vi "GUI_HTU_Vacuum.vi"() -> ()   [LabVIEW 2020]
uses:
  Shared/GUI_Template/GUI_master/tcp_new_data_event.ctl
  Shared/GUI_Template/GUI_master/tcp new data cluster.ctl
panel:
  out "AI_mean.Channel 3::1":dbl caption="Energy (nJ)" min=0.0 max=0.0 format="%.3f"
  out "AI_mean.Channel 2::1":dbl caption="Energy (nJ)" min=0.0 max=0.0 format="%.3f"
  out "highPressure 4":bool=TRUE
  out "highPressure 3":bool=TRUE
  out "Compressor":dbl format="%_6g"
  out "OAP":dbl
  out "highPressure 2":bool=TRUE
  out "highPressure":bool=TRUE
  in  "GUIdevice 2":string="U_DG645_ShotControl"
  out "TargetChamberP":dbl format="%_6g"
  out "UndulatorP":dbl
  out "AI_mean.Channel 1::1":dbl caption="Energy (nJ)" min=0.0 max=0.0 format="%.3f"
  out "AI_mean.Channel 0::1":dbl caption="Energy (nJ)" min=0.0 max=0.0 format="%.3f"
  in  "UDP error message":string
  in  "GUIdevice 1":string="U_VacuumGauge"
  out "error IO 2":errorcluster
  out "tcp data event":T1
  in  "stop":bool
  out "Chart":T2(graph)
  # "HTU Vacuum"
  # "Pressure (Torr)"
  # "Comp chamber"
  # "OAP chamber"
  # "Target chamber"
  # "A-cave"
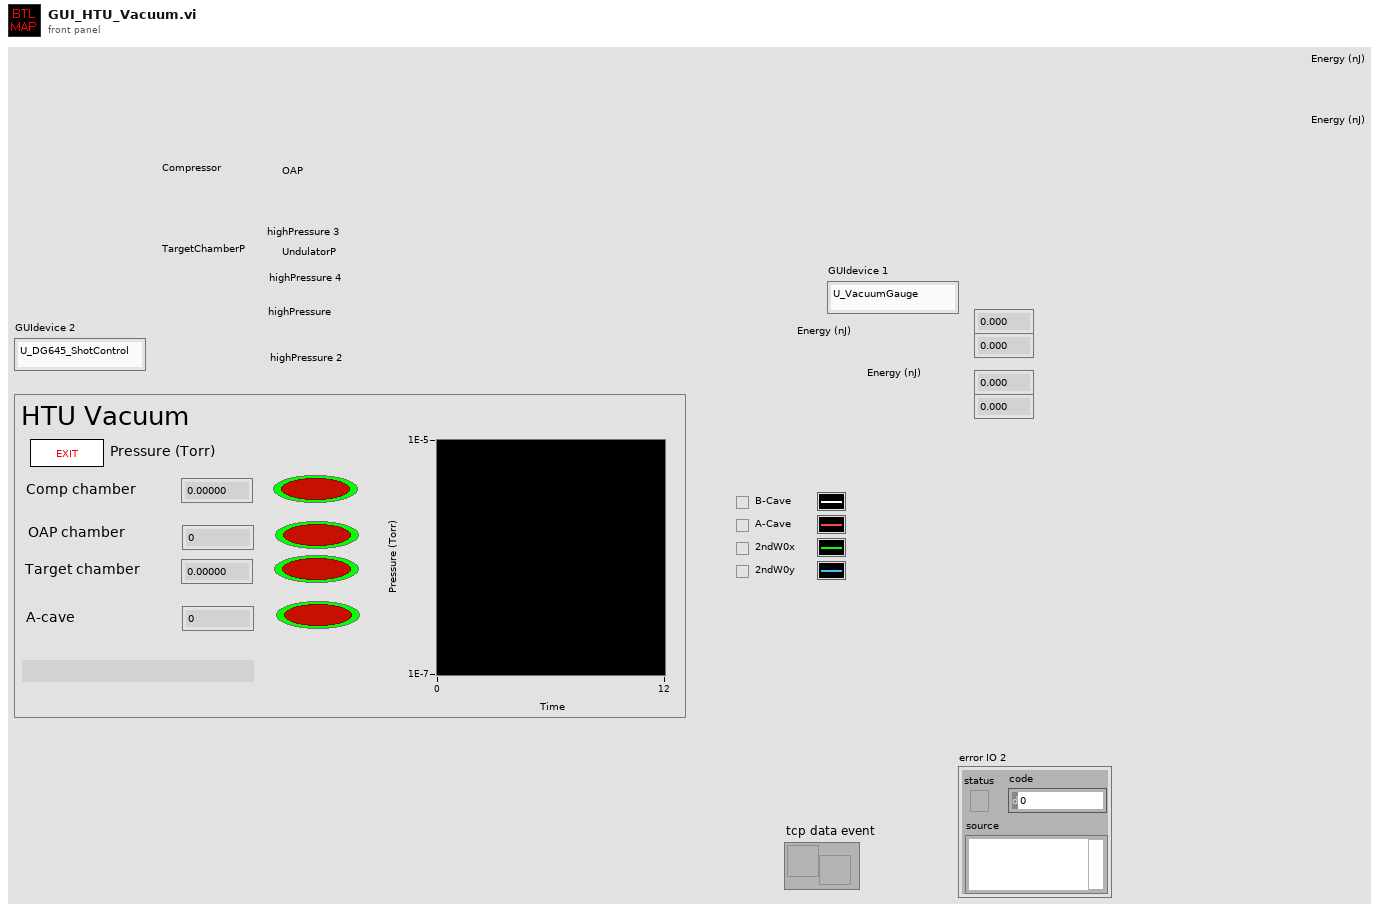
[diagram p1: front panel]
types:
  T1 = typedef "tcp_new_data_event.ctl" = refnum<user-event>
  T2 = cluster{"output variable":dbl, "output variable":dbl, "output variable":dbl, "output variable":dbl}
  T3 = typedef "tcp new data cluster.ctl" = cluster{"EventEnum":enum16{"new data", "connection status update"}, "Device name":string}
  T4 = enum32{"invalid app kind", "Development System", "Run Time System", "Student Edition", "Embedded LabVIEW", "Evaluation", "Custom"}
  T5 = enum32{"Invalid", "Standard", "Closed", "Hidden", "Minimized", "Maximized"}
  T6 = cluster{"Core":cluster{"Current VI Reference":refnum<vi>, "Close Panel on Exit?":bool}, "last chart update tck":i32, "TargetChamber":dbl, "Undulator":dbl, "CompressorChamber":dbl, "OAPChamber":dbl}
  T7 = cluster{"Current VI Reference":refnum<vi>, "Close Panel on Exit?":bool}
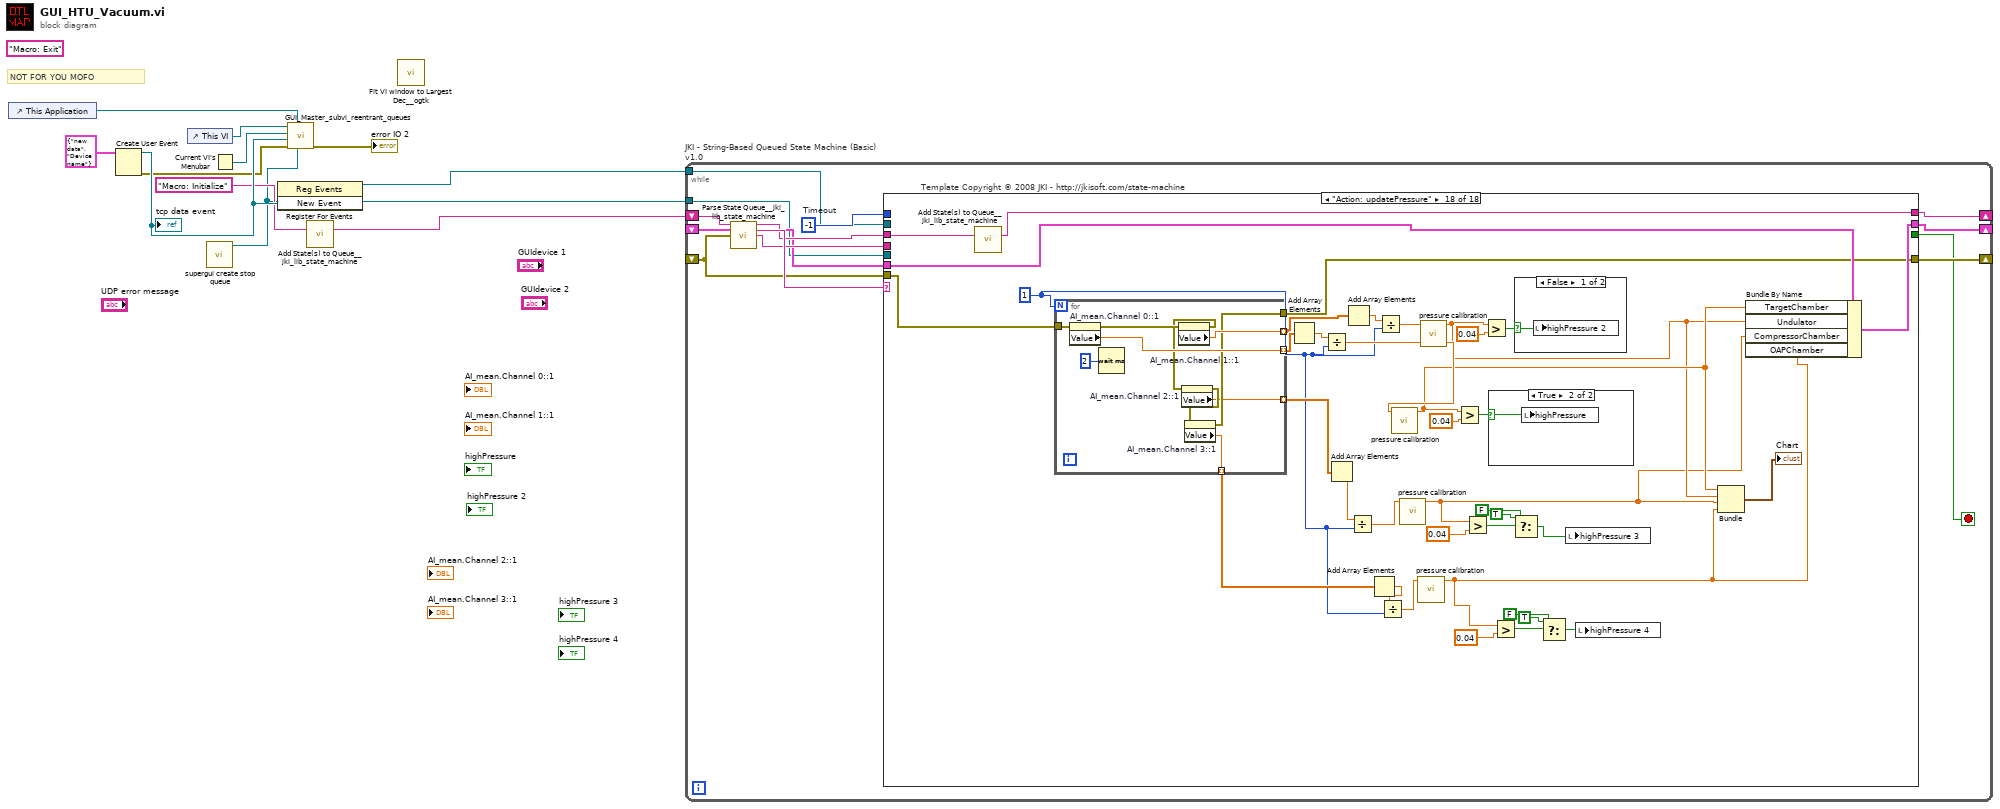
[diagram p0: block diagram]
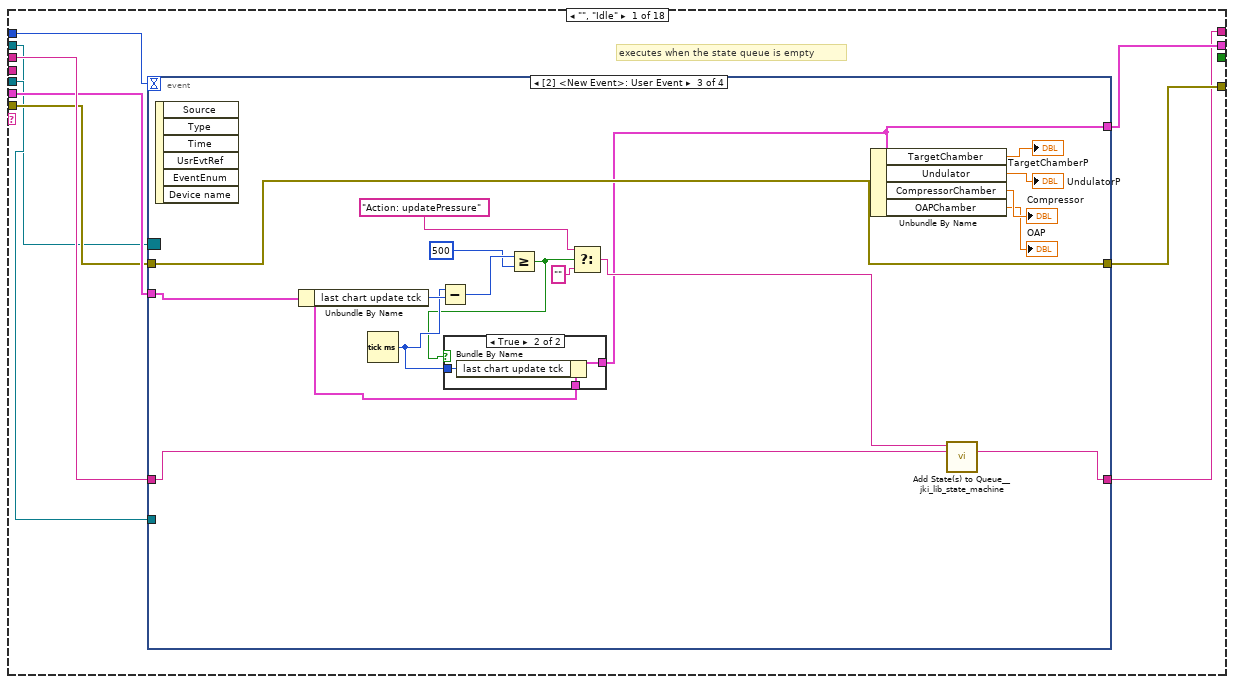
[diagram p2: hidden frame]
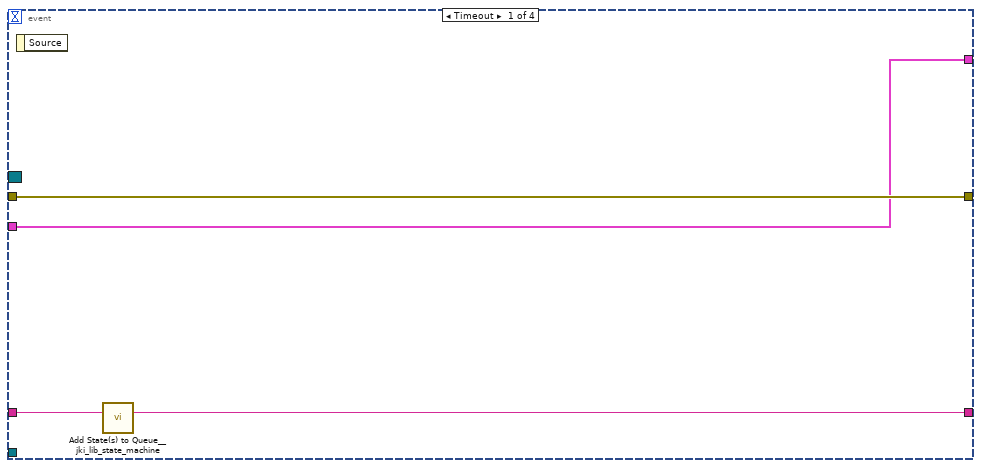
[diagram p3: hidden frame]
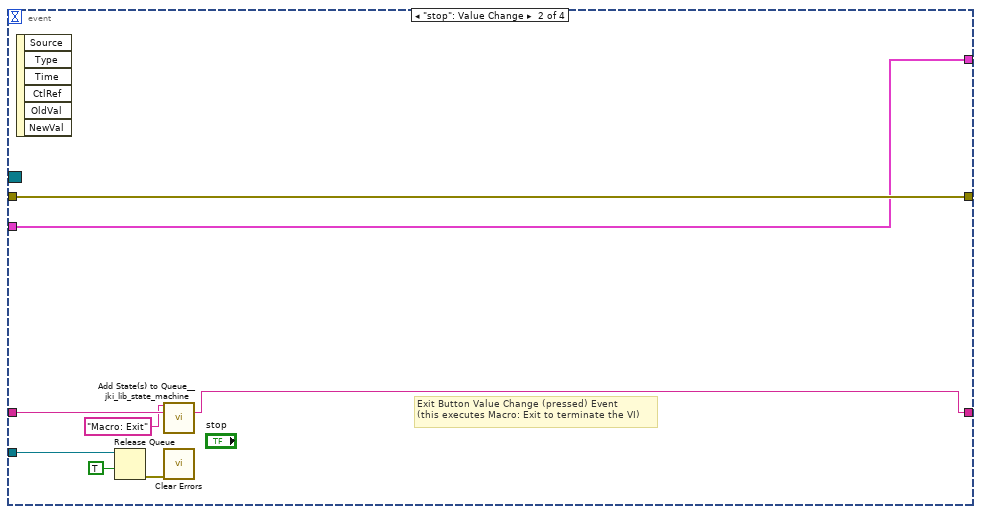
[diagram p4: hidden frame]
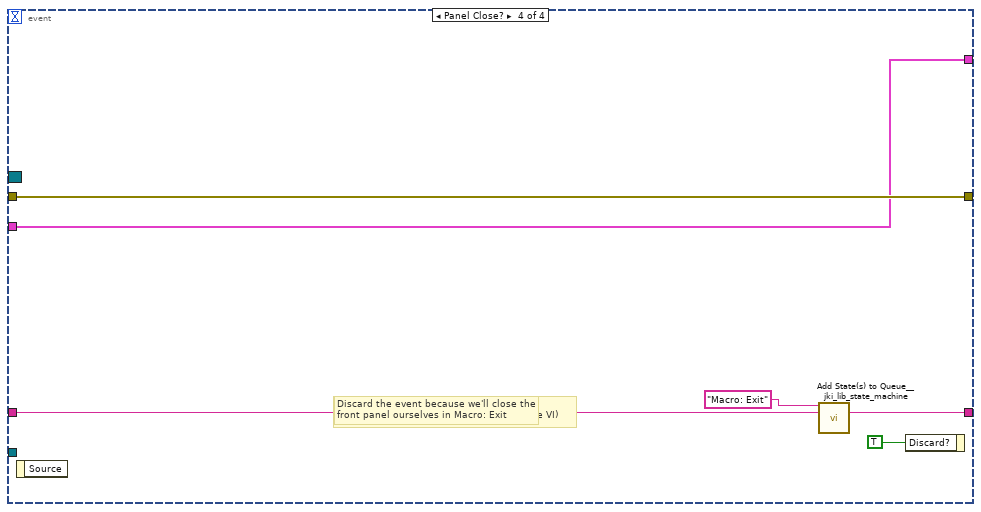
[diagram p6: hidden frame]
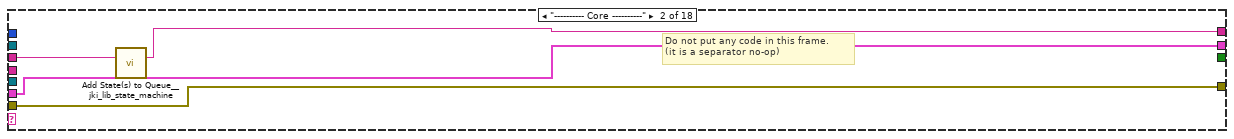
[diagram p7: hidden frame]
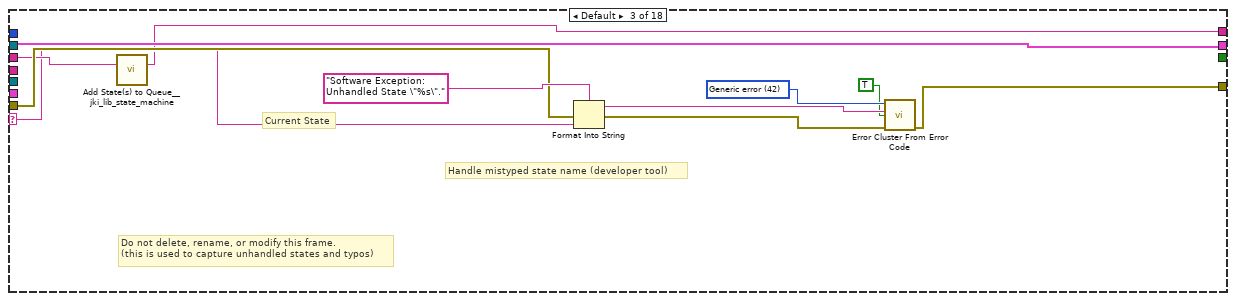
[diagram p8: hidden frame]
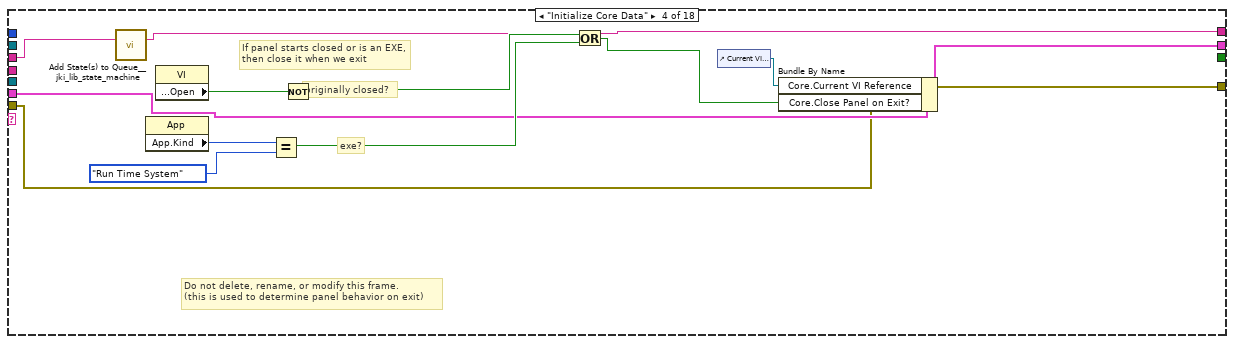
[diagram p9: hidden frame]
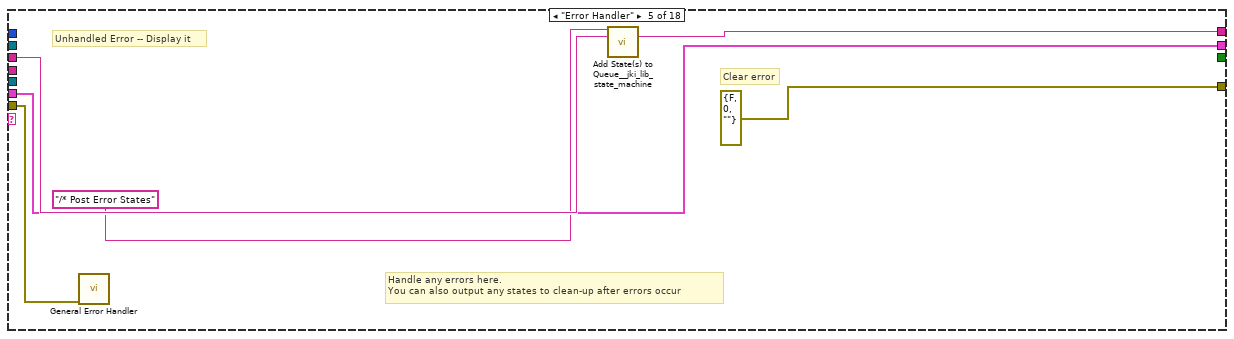
[diagram p10: hidden frame]
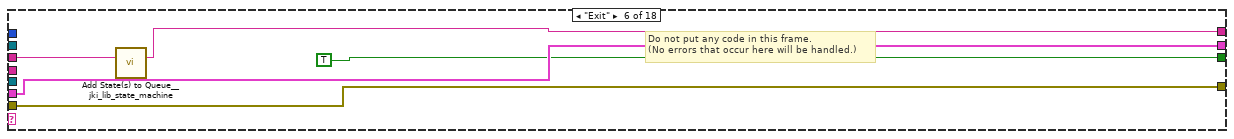
[diagram p11: hidden frame]
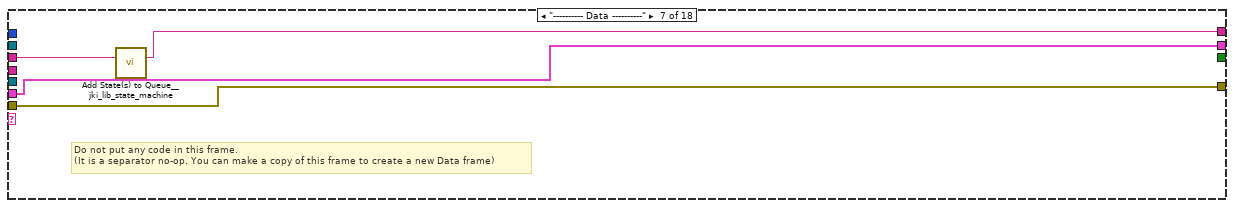
[diagram p12: hidden frame]
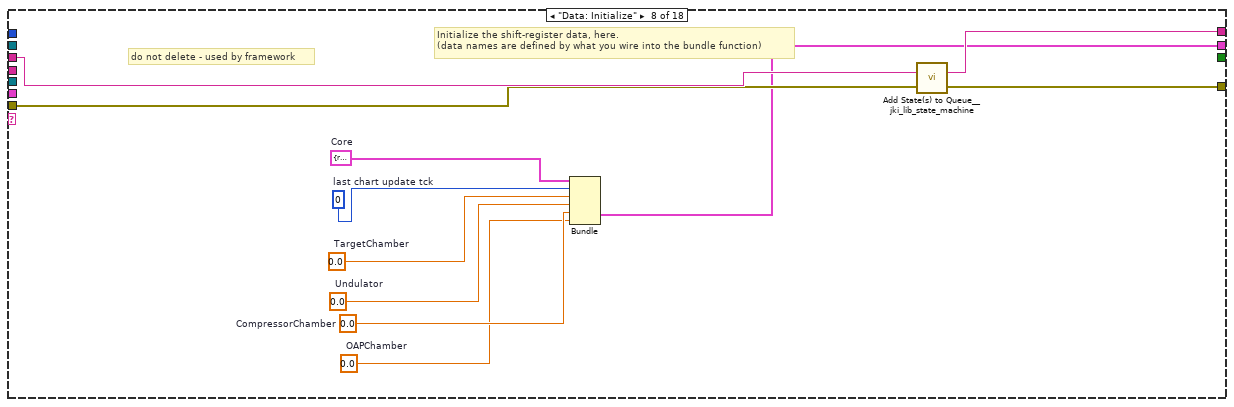
[diagram p13: hidden frame]
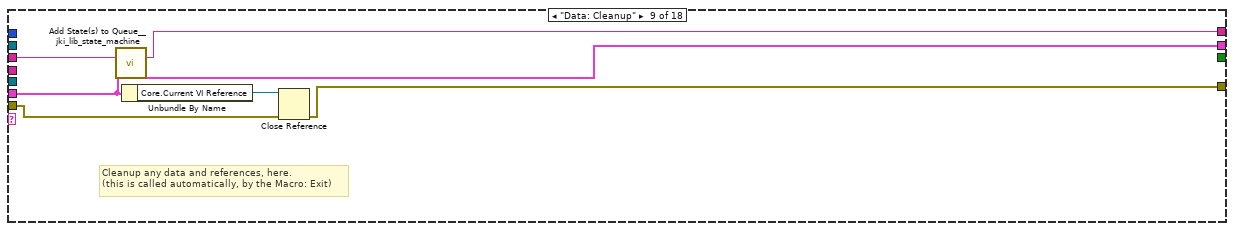
[diagram p14: hidden frame]
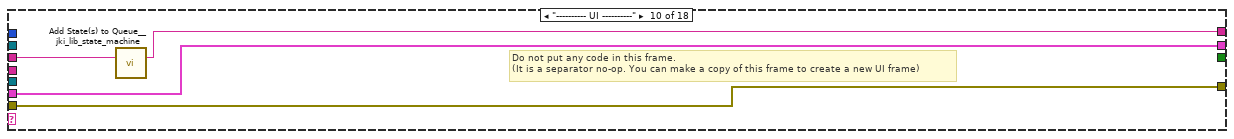
[diagram p15: hidden frame]
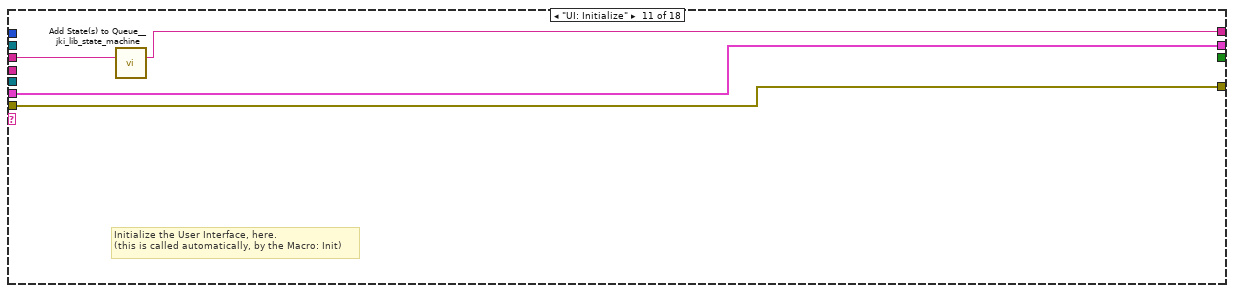
[diagram p16: hidden frame]
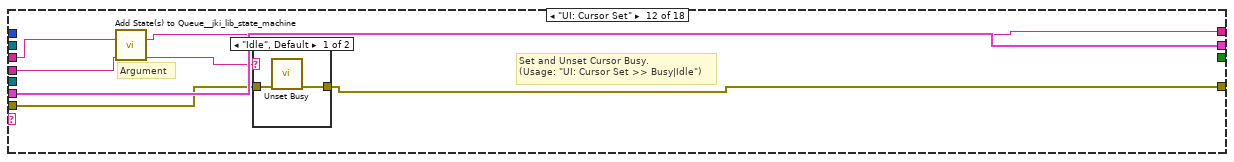
[diagram p17: hidden frame]
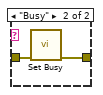
[diagram p18: hidden frame]
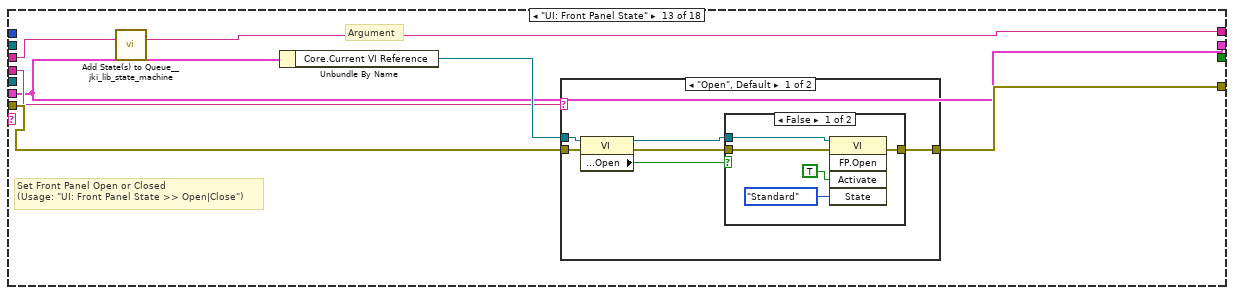
[diagram p19: hidden frame]
diagram:
  (unwired) "Macro: Exit"
  # "NOT FOR YOU MOFO"
  n1 = control-ref of="This Application"() -> (w11:refnum<vi>)
  n2 = Create User Event(user event datatype=T3 {"EventEnum"=enum."new data", "Device name"="Device name"} ("New Event")) -> (user event=w10:refnum<user-event>, error out=w9:errorcluster)  [unwired: 1 in]
  "tcp data event" <- w10
  n3 = control-ref of="This VI"() -> (w5:refnum<vi>)
  n4 = call "supergui create stop queue.vi"() -> ("STOP Queue out"=w1:refnum<queue>)  [unwired: 11 in]
  n5 = Current VI's Menubar() -> (w7:refnum<k9>)
  n6 = register-events(w10) -> (reference out=w2:refnum<event-registration>)  [unwired: 2 in, 1 out]
  n7 = call "GUI_Master_subvi_reentrant_queues.vi"("STOP Queue in"=w1, "This Application"=w11, "error in (no error)"=w9, "tcp data event"=w10, "Caller menu reference"=w7, "Caller VI ref"=w5) -> ("error out"=→"error IO 2":errorcluster)  [unwired: 5 in]
  n8 = call <vilib>:"Add State(s) to Queue__jki_lib_state_machine.vi"("State(s) in (\"\")"="Macro: Initialize") -> ("States Out"=w3:string)  [unwired: 14 in]
  n9 = call <userlib>:"Fit VI window to Largest Dec__ogtk.vi"() -> ()  [unwired: 6 in, 2 out]
  n10 = while "JKI - String-Based Queued State Machine (Basic) v1.0" {
    shift-right: [w18] -> _
    shift-left: _ -> [w17]
    shift-right: [w20] -> _
    shift-left: _ -> [w15]
    shift-right: [w12] -> _
    shift-left: w3 -> [w21]
    tunnel: w2 -> [w14]
    tunnel: w1 -> [w13]
    stop <- w19 stop-if-true
    w16 = -1  # Timeout
    # "Template Copyright © 2008 JKI - http://jkisoft.com/state-machine"
    n11 = call <vilib>:"Parse State Queue__jki_lib_state_machine.vi"("State Queue"=w21, "Error In (no error)"=w15) -> ("Remaining States"=w23:string, "Current State"=w24:string, "Arguments"=w22:string)  [unwired: 11 in]
    n12 = case shown="\"Action: updatePressure\"" w24 {
      selector: w24 -> [_ _ w78 _ _ _ _ _ _ _ _ _ _ _ _ _ _ _]
      tunnel: w23 -> [w33 w76 w81 w99 w105 w110 w114 w124 w130 w134 w138 w144 w155 w181 w186 w196 w200 w238]
      tunnel: w22 -> [_ _ _ _ _ _ _ _ _ _ _ w140 w151 _ _ _ _ _]
      tunnel: w17 -> [w32 w74 w80 w91 w104 w109 w112 _ w126 w132 w137 w143 w150 w179 w184 w188 w198 w236]
      tunnel: [w31 w75 w83 w88 errorcluster {"status"=FALSE, "code"=0, "source"=""} ("error out") w108 w113 w123 w128 w133 w136 w141 w153 w180 w185 w195 w199 w229] -> w20
      tunnel: w15 -> [w30 w75 w82 w88 w103 w108 w113 w123 w129 w133 w136 w142 w154 w180 w185 w195 w199 w230]
      tunnel: [_ _ _ _ _ TRUE _ _ _ _ _ _ _ _ _ _ _ _] -> w19
      tunnel: [w27 w74 w80 w90 w104 w109 w112 w120 w126 w132 w137 w143 w150 w179 w184 w188 w198 w235] -> w18
      tunnel: w16 -> [w29 _ _ _ _ _ _ _ _ _ _ _ _ _ _ _ _ _]
      tunnel: w14 -> [w25 _ _ _ _ _ _ _ _ _ _ _ _ _ _ _ _ _]
      tunnel: w13 -> [w28 _ _ _ _ _ _ _ _ _ _ _ _ _ _ _ _ _]
      tunnel: [w26 w73 w77 w89 w100 w106 w111 w121 w125 w131 w135 w139 w149 w178 w182 w187 w197 w237] -> w12
      frame "", "Idle" {
        # "executes when the state queue is empty"
        n13 = event shown="[2] <New Event>: User Event" {
          selector: w25 -> [_ _ _ _]
          dyn-events: _ -> [_ _ _ _]
          timeout: w29 -> [_ _ _ _]
          tunnel: w33 -> [w37 w45 w60 w72]
          tunnel: [w36 w44 w59 w71] -> w26
          tunnel: w32 -> [w34 w42 w61 w69]
          tunnel: [w35 w43 w62 w70] -> w31
          tunnel: w30 -> [w35 w43 w62 w70]
          tunnel: [w34 w42 w57 w69] -> w27
          tunnel: w28 -> [_ w39 _ _]
          event Timeout {
            n14 = event-data() -> ()  [unwired: 1 in, 1 out]
            n15 = call <vilib>:"Add State(s) to Queue__jki_lib_state_machine.vi"("State(s) in (\"\")"=w37) -> ("States Out"=w36:string)  [unwired: 14 in]
          }
          event "stop": Value Change {
            # "Exit Button Value Change (pressed) Event\n(this executes Macro: Exit to terminate the VI)"
            n16 = event-data() -> ()  [unwired: 1 in, 6 out]
            n17 = Release Queue(queue=w39, force destroy? (F)=TRUE) -> (error out=w40:errorcluster)  [unwired: 1 in, 2 out]
            n18 = call <vilib>:"Add State(s) to Queue__jki_lib_state_machine.vi"("State(s) in Front (\"\")"="Macro: Exit", "State(s) in (\"\")"=w45) -> ("States Out"=w44:string)  [unwired: 13 in]
            n19 = call <vilib>:"Clear Errors.vi"("error in (no error)"=w40) -> ()  [unwired: 5 in, 2 out]
          }
          event User Event {
            n20 = event-data() -> ()  [unwired: 1 in, 6 out]
            n21 = Unbundle By Name(w61) -> ("last chart update tck"=w55:i32)
            n22 = Tick Count (ms)() -> (millisecond timer value=w51:u32)
            n23 = Subtract(x=w51, y=w55) -> (x-y=w54:u32)
            n24 = Greater Or Equal?(x=w54, y=u32 500 ("x")) -> (x >= y?=w48:bool)
            n25 = case shown="True" w48 {
              tunnel: [w63 w66] -> w57
              tunnel: w61 -> [w63 w65]
              tunnel: w51 -> [_ w64]
              frame False {
              }
              frame True {
                n26 = Bundle By Name(cluster=w65, "last chart update tck"=w64) -> (w66:T6)
              }
            }
            n27 = Select(t="Action: updatePressure", s=w48, f="") -> (s? t:f=w58:string)
            n28 = Unbundle By Name(w57) -> ("TargetChamber"=→"TargetChamberP":dbl, "Undulator"=→"UndulatorP":dbl, "CompressorChamber"=→"Compressor":dbl, "OAPChamber"=→"OAP":dbl)
            n29 = call <vilib>:"Add State(s) to Queue__jki_lib_state_machine.vi"("State(s) in Front (\"\")"=w58, "State(s) in (\"\")"=w60) -> ("States Out"=w59:string)  [unwired: 13 in]
          }
          event Panel Close? {
            # "Discard the event because we'll close the front panel ourselves in Macro: Exit"
            # "Close Panel button (pressed) Event\n(this executes Macro: Exit to terminate the VI)"
            n30 = event-data() -> ()  [unwired: 1 in, 1 out]
            n31 = call <vilib>:"Add State(s) to Queue__jki_lib_state_machine.vi"("State(s) in Front (\"\")"="Macro: Exit", "State(s) in (\"\")"=w72) -> ("States Out"=w71:string)  [unwired: 13 in]
            n32 = event-data("Discard?"=TRUE) -> ()  [unwired: 1 in, 1 out]
          }
        }
      }
      frame "---------- Core ----------" {
        # "Do not put any code in this frame.\n(it is a separator no-op)"
        n33 = call <vilib>:"Add State(s) to Queue__jki_lib_state_machine.vi"("State(s) in (\"\")"=w76) -> ("States Out"=w73:string)  [unwired: 14 in]
      }
      frame Default {
        w86 = 42 items=["No error", "Argument error", "Memory is full", "Out of zone", "End of file", "File already open", "Generic file I/O error", "File not found", "File permission error", "Disk is full", "Duplicate path", "Too many files open", "System feature not enabled", "Resource file not found", "Cannot add resource", "Resource not found", "Image not found", "Image memory error", "Pen does not exist", "Config type invalid", "Config token not found", "Config parse error", "Config memory error", "Bad external code format", "Bad external code offset", "External code not present", "Null window", "Destroy window error", "Null menu", "Print aborted", "Bad print record", "Print driver error", "Windows error during printing", "Memory error during printing", "Print dialog error", "Generic print error", "Invalid device refnum", "Device not found", "Device parameter error", "Device unit error", "Cannot open device", "Device call aborted", "Generic error", "Cancelled by user", "Object ID too low", "Object ID too high", "Object not in heap", "Unknown heap", "Unknown object (invalid DefProc)", "Unknown object (DefProc not in table)", "Message out of range", "Invalid (null) method", "Unknown message", "Manager call not supported", "Bad address", "Network operation in progress", "Network operation timed out", "Connection is busy", "Network attribute not supported", "Network error", "Address in use", "System out of memory", "Connection aborted", "Connection refused", "Not connected", "Already connected", "Connection closed", "Initialization error (interapplication manager)", "Bad occurrence", "Wait on unbound occurrence handler", "Occurrence queue overflow", "Datalog type conflict", "Unused", "Unrecognized type (interapplication manager)", "Memory corrupt", "Failed to make temporary DLL", "Old CIN version", "Drag socket not found", "Failed to load drop-object", "Failed to register OLE object", "Failed to release OLE object", "Format specifier type mismatch", "Unknown format specifier", "Too few format specifiers", "Too many format specifiers", "Scan failed", "Newer CIN version", "Error converting to variant", "Runtime menu error", "Password tampered", "Variant attribute not found", "Incompatible variant data type", "Event data is not available", "Event Store is not present", "Occurrence is not found", "Event Queue is not created", "Event info is not available", "Refnum passed is NULL", "Error retrieving Class GUID", "Error retrieving CoClass GUID", "Error retrieving TypeLib GUID.", "Bad built application magic bytes.", "Specific driver is different from the specific driver associated with the Logical Name.", "There is no session opened to the class driver.", "Max Error", "MAX - Error with config objects", "MAX - Error loading configuration", "MAX - Group not supported"]
        # "Current State"
        # "Do not delete, rename, or modify this frame.\n(this is used to capture unhandled states and typos)"
        # "Handle mistyped state name (developer tool)"
        n34 = call <vilib>:"Add State(s) to Queue__jki_lib_state_machine.vi"("State(s) in (\"\")"=w81) -> ("States Out"=w77:string)  [unwired: 14 in]
        n35 = Format Into String(format string="Software Exception: Unhandled State \"%s\"." ("message"), error in=w82, w78) -> (resulting string=w85:string, error out=w84:errorcluster)  [unwired: 1 in]
        n36 = call <vilib>:"Error Cluster From Error Code.vi"("show call chain? (False)"=TRUE, "error in (no error)"=w84, "error message (\"\")"=w85, "error code (0)"=w86) -> ("error out"=w83:errorcluster)  [unwired: 5 in]
      }
      frame "Initialize Core Data" {
        # "Do not delete, rename, or modify this frame.\n(this is used to determine panel behavior on exit)"
        # "originally closed?"
        # "exe?"
        # "If panel starts closed or is an EXE, then close it when we exit"
        n37 = call <vilib>:"Add State(s) to Queue__jki_lib_state_machine.vi"("State(s) in (\"\")"=w99) -> ("States Out"=w89:string)  [unwired: 14 in]
        n38 = property class="App"() -> ("App.Kind"=w97:T4)  [unwired: 2 in, 2 out]
        n39 = property class="VI"() -> ("Front Panel.Open"=w98:bool)  [unwired: 2 in, 2 out]
        n40 = Equal?(x=w97, y=T4."Run Time System" ("Application:Kind")) -> (x = y?=w94:bool)
        n41 = Not(x=w98) -> (.not. x?=w95:bool)
        n42 = Or(x=w95, y=w94) -> (x .or. y?=w93:bool)
        n43 = control-ref of="Current VI Reference"() -> (w92:refnum<vi>)
        n44 = Bundle By Name(cluster=w91, "Core.Current VI Reference"=w92, "Core.Close Panel on Exit?"=w93) -> (w90:T6)
      }
      frame "Error Handler" {
        # "Unhandled Error -- Display it"
        # "Handle any errors here.\nYou can also output any states to clean-up after errors occur"
        # "Clear error"
        n45 = call <vilib>:"General Error Handler.vi"("error in (no error)"=w103) -> ()  [unwired: 10 in, 5 out]
        n46 = call <vilib>:"Add State(s) to Queue__jki_lib_state_machine.vi"("State(s) in Front (\"\")"="/* Post Error States", "State(s) in (\"\")"=w105) -> ("States Out"=w100:string)  [unwired: 13 in]
      }
      frame "Exit" {
        # "Do not put any code in this frame.\n(No errors that occur here will be handled.)"
        n47 = call <vilib>:"Add State(s) to Queue__jki_lib_state_machine.vi"("State(s) in (\"\")"=w110) -> ("States Out"=w106:string)  [unwired: 14 in]
      }
      frame "---------- Data ----------" {
        # "Do not put any code in this frame.\n(It is a separator no-op. You can make a copy of this frame to create a new Data frame)"
        n48 = call <vilib>:"Add State(s) to Queue__jki_lib_state_machine.vi"("State(s) in (\"\")"=w114) -> ("States Out"=w111:string)  [unwired: 14 in]
      }
      frame "Data: Initialize" {
        w115 = 0.0  # OAPChamber
        w116 = 0.0  # CompressorChamber
        w117 = 0.0  # Undulator
        w118 = 0.0  # TargetChamber
        w119 = 0  # last chart update tck
        w122 = T7 {"Current VI Reference"=refnum, "Close Panel on Exit?"=FALSE}  # Core
        # "do not delete - used by framework"
        # "Initialize the shift-register data, here.\n(data names are defined by what you wire into the bundle function)"
        n49 = Bundle("Core"=w122, "last chart update tck"=w119, "TargetChamber"=w118, "Undulator"=w117, "CompressorChamber"=w116, "OAPChamber"=w115) -> (w120:T6)  [unwired: 1 in]
        n50 = call <vilib>:"Add State(s) to Queue__jki_lib_state_machine.vi"("State(s) in (\"\")"=w124) -> ("States Out"=w121:string)  [unwired: 14 in]
      }
      frame "Data: Cleanup" {
        # "Cleanup any data and references, here.\n(this is called automatically, by the Macro: Exit)"
        n51 = call <vilib>:"Add State(s) to Queue__jki_lib_state_machine.vi"("State(s) in (\"\")"=w130) -> ("States Out"=w125:string)  [unwired: 14 in]
        n52 = Unbundle By Name(w126) -> ("Core.Current VI Reference"=w127:refnum<vi>)
        n53 = Close Reference(reference=w127, error in (no error)=w129) -> (error out=w128:errorcluster)
      }
      frame "---------- UI ----------" {
        # "Do not put any code in this frame.\n(It is a separator no-op. You can make a copy of this frame to create a new UI frame)"
        n54 = call <vilib>:"Add State(s) to Queue__jki_lib_state_machine.vi"("State(s) in (\"\")"=w134) -> ("States Out"=w131:string)  [unwired: 14 in]
      }
      frame "UI: Initialize" {
        # "Initialize the User Interface, here.\n(this is called automatically, by the Macro: Init)"
        n55 = call <vilib>:"Add State(s) to Queue__jki_lib_state_machine.vi"("State(s) in (\"\")"=w138) -> ("States Out"=w135:string)  [unwired: 14 in]
      }
      frame "UI: Cursor Set" {
        # "Argument"
        # "Set and Unset Cursor Busy.\n(Usage: \"UI: Cursor Set >> Busy|Idle\")"
        n56 = call <vilib>:"Add State(s) to Queue__jki_lib_state_machine.vi"("State(s) in (\"\")"=w144) -> ("States Out"=w139:string)  [unwired: 14 in]
        n57 = case shown="\"Idle\", Default" w140 {
          tunnel: w142 -> [w146 w148]
          tunnel: [w145 w147] -> w141
          frame "Idle", Default {
            n58 = call <vilib>:"Unset Busy.vi"("error in (no error)"=w146) -> ("error out"=w145:errorcluster)  [unwired: 10 in]
          }
          frame "Busy" {
            n59 = call <vilib>:"Set Busy.vi"("error in (no error)"=w148) -> ("error out"=w147:errorcluster)  [unwired: 9 in, 1 out]
          }
        }
      }
      frame "UI: Front Panel State" {
        # "Argument"
        # "Set Front Panel Open or Closed\n(Usage: \"UI: Front Panel State >> Open|Close\")"
        n60 = call <vilib>:"Add State(s) to Queue__jki_lib_state_machine.vi"("State(s) in (\"\")"=w155) -> ("States Out"=w149:string)  [unwired: 14 in]
        n61 = Unbundle By Name(w150) -> ("Core.Current VI Reference"=w152:refnum<vi>)
        n62 = case shown="\"Open\", Default" w151 {
          tunnel: w154 -> [w160 w172]
          tunnel: [w161 w173] -> w153
          tunnel: w152 -> [w156 w168]
          frame "Open", Default {
            n63 = property class="VI"(reference=w156, error in=w160) -> (reference out=w158:refnum<vi>, error out=w159:errorcluster, "Front Panel.Open"=w157:bool)
            n64 = case shown="False" w157 {
              tunnel: [w164 w167] -> w161
              tunnel: w159 -> [w163 w167]
              tunnel: w158 -> [w162 _]
              frame False {
                n65 = invoke class="VI" method="FP.Open"(reference=w162, error in=w163, "Activate"=TRUE, "State"=T5."Standard") -> (error out=w164:errorcluster)  [unwired: 1 in, 4 out]
              }
              frame True {
              }
            }
          }
          frame "Close" {
            n66 = property class="VI"(reference=w168, error in=w172) -> (reference out=w170:refnum<vi>, error out=w171:errorcluster, "Front Panel.Open"=w169:bool)
            n67 = case shown="True" w169 {
              tunnel: [w174 w177] -> w173
              tunnel: w171 -> [w174 w176]
              tunnel: w170 -> [_ w175]
              frame False {
              }
              frame True {
                n68 = invoke class="VI" method="FP.Close"(reference=w175, error in=w176) -> (error out=w177:errorcluster)  [unwired: 1 in, 2 out]
              }
            }
          }
        }
      }
      frame "---------- Macro ----------" {
        # "Do not put any code in this frame.\n(It is a separator no-op. You can make a copy of this frame to create a new Macro frame)"
        n69 = call <vilib>:"Add State(s) to Queue__jki_lib_state_machine.vi"("State(s) in (\"\")"=w181) -> ("States Out"=w178:string)  [unwired: 14 in]
      }
      frame "Macro: Initialize" {
        w183 = "Data: Initialize\nInitialize Core Data\nUI: Initialize\nUI: Front Panel State >> Open"  # Data: Initialize Initialize Core Data UI: Initialize UI: Front Panel State >> Open
        # "Initialization Macro\n(This is called once, when the VI starts)"
        n70 = call <vilib>:"Add State(s) to Queue__jki_lib_state_machine.vi"("State(s) in Front (\"\")"=w183, "State(s) in (\"\")"=w186) -> ("States Out"=w182:string)  [unwired: 13 in]
      }
      frame "Macro: Exit" {
        # "Exit Macro\n(This is called once, when the VI exits)"
        n71 = Unbundle By Name(w188) -> ("Core.Close Panel on Exit?"=w189:bool)
        n72 = Select(t="UI: Front Panel State >> Close", s=w189, f="") -> (s? t:f=w192:string)
        n73 = call <vilib>:"Add State(s) to Queue__jki_lib_state_machine.vi"("State(s) in (\"\")"=w192, "State(s) at Back (\"\")"="Data: Cleanup\nExit") -> ("States Out"=w190:string)  [unwired: 13 in]
        n74 = call <vilib>:"Add State(s) to Queue__jki_lib_state_machine.vi"("State(s) in Front (\"\")"=w190, "State(s) in (\"\")"=w196) -> ("States Out"=w187:string)  [unwired: 13 in]
      }
      frame "---------- New Category ----------" {
        n75 = call <vilib>:"Add State(s) to Queue__jki_lib_state_machine.vi"("State(s) in (\"\")"=w200) -> ("States Out"=w197:string)  [unwired: 14 in]
      }
      frame "Action: updatePressure" {
        w215 = 1
        n76 = call <vilib>:"Add State(s) to Queue__jki_lib_state_machine.vi"("State(s) in (\"\")"=w238) -> ("States Out"=w237:string)  [unwired: 14 in]
        n77 = for {
          N: w215 -> [_]
          tunnel: w230 -> [w247]
          tunnel: [w241] -> w229
          tunnel: [w246] -> w228 mode=indexing
          tunnel: [w245] -> w224 mode=indexing
          tunnel: [w240] -> w219 mode=indexing
          tunnel: [w239] -> w218 mode=indexing
          n78 = property on="AI_mean.Channel 0::1" class="DigNum (strict)"(error in=w247) -> (error out=w248:errorcluster, "Value"=w246:dbl)  [unwired: 1 in, 1 out]
          n79 = Wait (ms)(milliseconds to wait=u32 2) -> ()  [unwired: 1 out]
          n80 = property on="AI_mean.Channel 1::1" class="DigNum (strict)"(error in=w248) -> (error out=w243:errorcluster, "Value"=w245:dbl)  [unwired: 1 in, 1 out]
          n81 = property on="AI_mean.Channel 2::1" class="DigNum (strict)"(error in=w243) -> (error out=w242:errorcluster, "Value"=w240:dbl)  [unwired: 1 in, 1 out]
          n82 = property on="AI_mean.Channel 3::1" class="DigNum (strict)"(error in=w242) -> (error out=w241:errorcluster, "Value"=w239:dbl)  [unwired: 1 in, 1 out]
        }
        n83 = Add Array Elements(numeric array=w228) -> (sum=w227:dbl)
        n84 = Divide(x=w227, y=w215) -> (x/y=w226:dbl)
        n85 = Add Array Elements(numeric array=w219) -> (sum=w217:dbl)
        n86 = Add Array Elements(numeric array=w224) -> (sum=w225:dbl)
        n87 = Divide(x=w217, y=w215) -> (x/y=w216:dbl)
        n88 = Add Array Elements(numeric array=w218) -> (sum=w214:dbl)
        n89 = Divide(x=w225, y=w215) -> (x/y=w223:dbl)
        n90 = Divide(x=w214, y=w215) -> (x/y=w213:dbl)
        n91 = call "pressure calibration.vi"("input variable"=w226) -> ("output variable"=w221:dbl)  [unwired: 10 in]
        n92 = call "pressure calibration.vi"("input variable"=w216) -> ("output variable"=w212:dbl)  [unwired: 10 in]
        n93 = call "pressure calibration.vi"("input variable"=w213) -> ("output variable"=w202:dbl)  [unwired: 10 in]
        n94 = call "pressure calibration.vi"("input variable"=w223) -> ("output variable"=w220:dbl)  [unwired: 10 in]
        n95 = Greater?(x=w221, y=0.04) -> (0:w233:bool)
        n96 = Greater?(x=w212, y=0.04) -> (0:w210:bool)
        n97 = Greater?(x=w220, y=0.04) -> (0:w231:bool)
        n98 = case shown="True" w233 {
          selector: w233 -> [w251 w252]
          frame False {
            n99 = local write "highPressure"(w251) -> ()
          }
          frame True {
            n100 = local write "highPressure"(w252) -> ()
          }
        }
        n101 = Greater?(x=w202, y=0.04) -> (0:w205:bool)
        n102 = Select(t=TRUE, s=w210, f=FALSE) -> (s? t:f=w208:bool)
        n103 = case shown="False" w231 {
          selector: w231 -> [w249 w250]
          frame False {
            n104 = local write "highPressure 2"(w249) -> ()
          }
          frame True {
            n105 = local write "highPressure 2"(w250) -> ()
          }
        }
        n106 = Select(t=TRUE, s=w205, f=FALSE) -> (s? t:f=w201:bool)
        n107 = local write "highPressure 3"(w208) -> ()
        n108 = local write "highPressure 4"(w201) -> ()
        n109 = Bundle("output variable"=w221, "output variable"=w220, "output variable"=w212, "output variable"=w202) -> (→"Chart":T2)  [unwired: 1 in]
        n110 = Bundle By Name(cluster=w236, "TargetChamber"=w221, "Undulator"=w220, "CompressorChamber"=w212, "OAPChamber"=w202) -> (w235:T6)
      }
    }
  }
